vi "main_interface.vi"() -> ()   [LabVIEW 2019]
uses:
  <vilib>/Utility/miscctls.llb/LVPositionTypeDef.ctl
  <vilib>/DAQmx/read.llb/DAQmx Read (Analog 2D DBL NChan NSamp).vi
  <vilib>/DAQmx/miscellaneous.llb/DAQmx Fill In Error Info.vi
  <vilib>/Utility/file.llb/Write Delimited Spreadsheet (DBL).vi
  <vilib>/DAQmx/configure/timing.llb/DAQmx Timing (Sample Clock).vi
  <resource>/objmgr/daqmx.rc
panel:
  out "Actual Sample Rate":dbl=1000.0 format="%0.2f"
  in  "Sample Rate":dbl=3000.0
  in  "task/channels in":refnum<k21>="ADQUIRE"
  in  "PosProcessamento Button":bool
  out "Status Bar":string
  in  "Variaveis Button":bool
  in  "Home Button":bool
  in  "Calibracao Button":bool
  in  "[ESC]":bool
  in  "Tab Main":T1(tab)
  in  "Graph-PlotView-All":bool
  in  "Graph-PlotView-C":bool
  in  "Graph-PlotView-Pressoes":bool
  in  "Nome do Arquivo":string
  out "NI on?":bool
  in  "Start NI":bool
  out "aquisicao?":bool
  in  "Tempo Aquisicao":dbl
  in  "Start Aquisition":bool
  out "Dados NI [mA*10^-3]":dbl[](array[numeric])
  out "Pressoes [kPa]":dbl[](array[numeric])
  out "C Graph":dbl[][](graph)
  in  "calib_save_new":bool
  out "calib_max_atual P 11":dbl
  out "calib_min_atual P 11":dbl
  out "calib_max_atual P 10":dbl
  out "calib_min_atual P 10":dbl
  out "calib_max_atual P 9":dbl
  out "calib_min_atual P 9":dbl
  out "calib_max_atual P 8":dbl
  out "calib_min_atual P 8":dbl
  out "calib_max_atual P 7":dbl
  out "calib_min_atual P 7":dbl
  out "calib_max_atual P 6":dbl
  out "calib_min_atual P 6":dbl
  out "calib_max_atual P 5":dbl
  out "calib_min_atual P 5":dbl
  out "calib_max_atual P 4":dbl
  out "calib_min_atual P 4":dbl
  out "calib_max_atual P 3":dbl
  out "calib_min_atual P 3":dbl
  out "calib_max_atual P 2":dbl
  out "calib_min_atual P 2":dbl
  out "calib_max_atual P 1":dbl
  out "calib_min_atual P 1":dbl
  in  "calib_max_new P9":dbl
  in  "calib_min_new P9":dbl
  in  "calib_max_new P8":dbl
  in  "calib_min_new P8":dbl
  in  "calib_max_new P7":dbl
  in  "calib_min_new P7":dbl
  in  "calib_max_new P6":dbl
  in  "calib_min_new P6":dbl
  in  "calib_max_new P5":dbl
  in  "calib_min_new P5":dbl
  in  "calib_max_new P4":dbl
  in  "calib_min_new P4":dbl
  in  "calib_max_new P11":dbl
  in  "calib_min_new P11":dbl
  in  "calib_max_new P10":dbl
  in  "calib_min_new P10":dbl
  in  "calib_max_new P3":dbl
  in  "calib_min_new P3":dbl
  in  "calib_max_new P2":dbl
  in  "calib_min_new P2":dbl
  in  "calib_max_new P1":dbl
  in  "calib_min_new P1":dbl
  out "dat files":string[](array[string])
  in  "Open Folder DAT":bool
  in  "posProcessamento_button_all":bool
  in  "posProcessamento_button_indv":bool
  in  "Read TDMS file":bool
  in  "path_posProcessamento":path
  out "size dat dir":i64
  in  "Tempo aux":dbl
  out "Tempo Decorrido":dbl
  in  "Brilho do botao NI":bool
  # "Adquiri \nLazyWave"
  # "Tempo de Aquisição [s]"
  # "*Dados coletados diretamente da placa NI,\npodem estar fora de escala"
  # "Calibração atual"
  # "Nova calibração"
  # "P1"
  # "P2"
  # "P3"
  # "P4"
  # "P5"
  # "P6"
  # "P7"
  # "P8"
  # "P9"
  # "P10"
  # "P11"
  # "Arquivos processados"
  # "Processamento de um arquivo"
  # "Abrir arquivo TDMS"
  # "Abrir pasta com os arquivos .DAT"
  # "Processar todos os arquivos"
  # "Directory size"
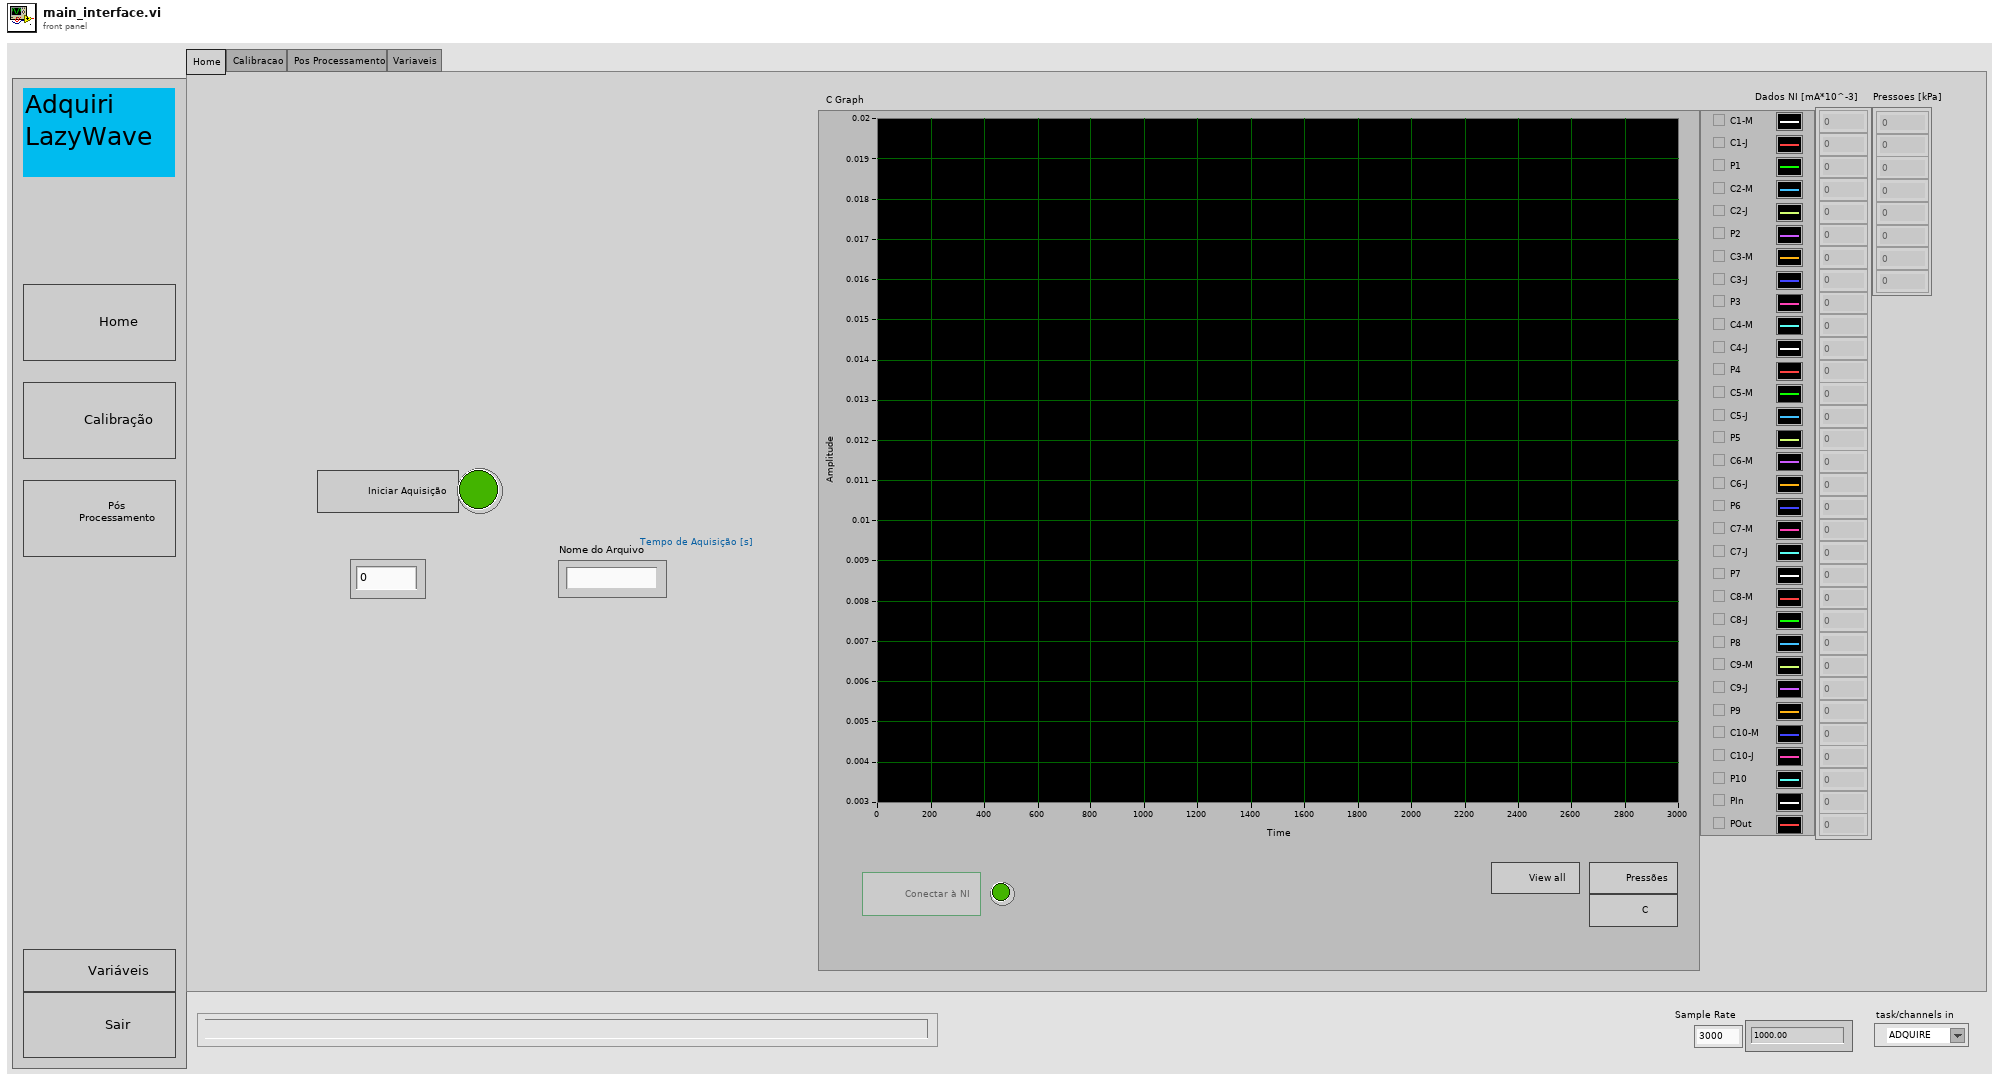
[diagram p1: front panel]
types:
  T1 = enum32{"Home", "Calibracao", "Pos Processamento", "Variaveis"}
  T2 = enum8{"Enabled", "Disabled", "Disabled and Grayed Out"}
  T3 = typedef "LVPositionTypeDef.ctl" = cluster{"Left":i32, "Top":i32}
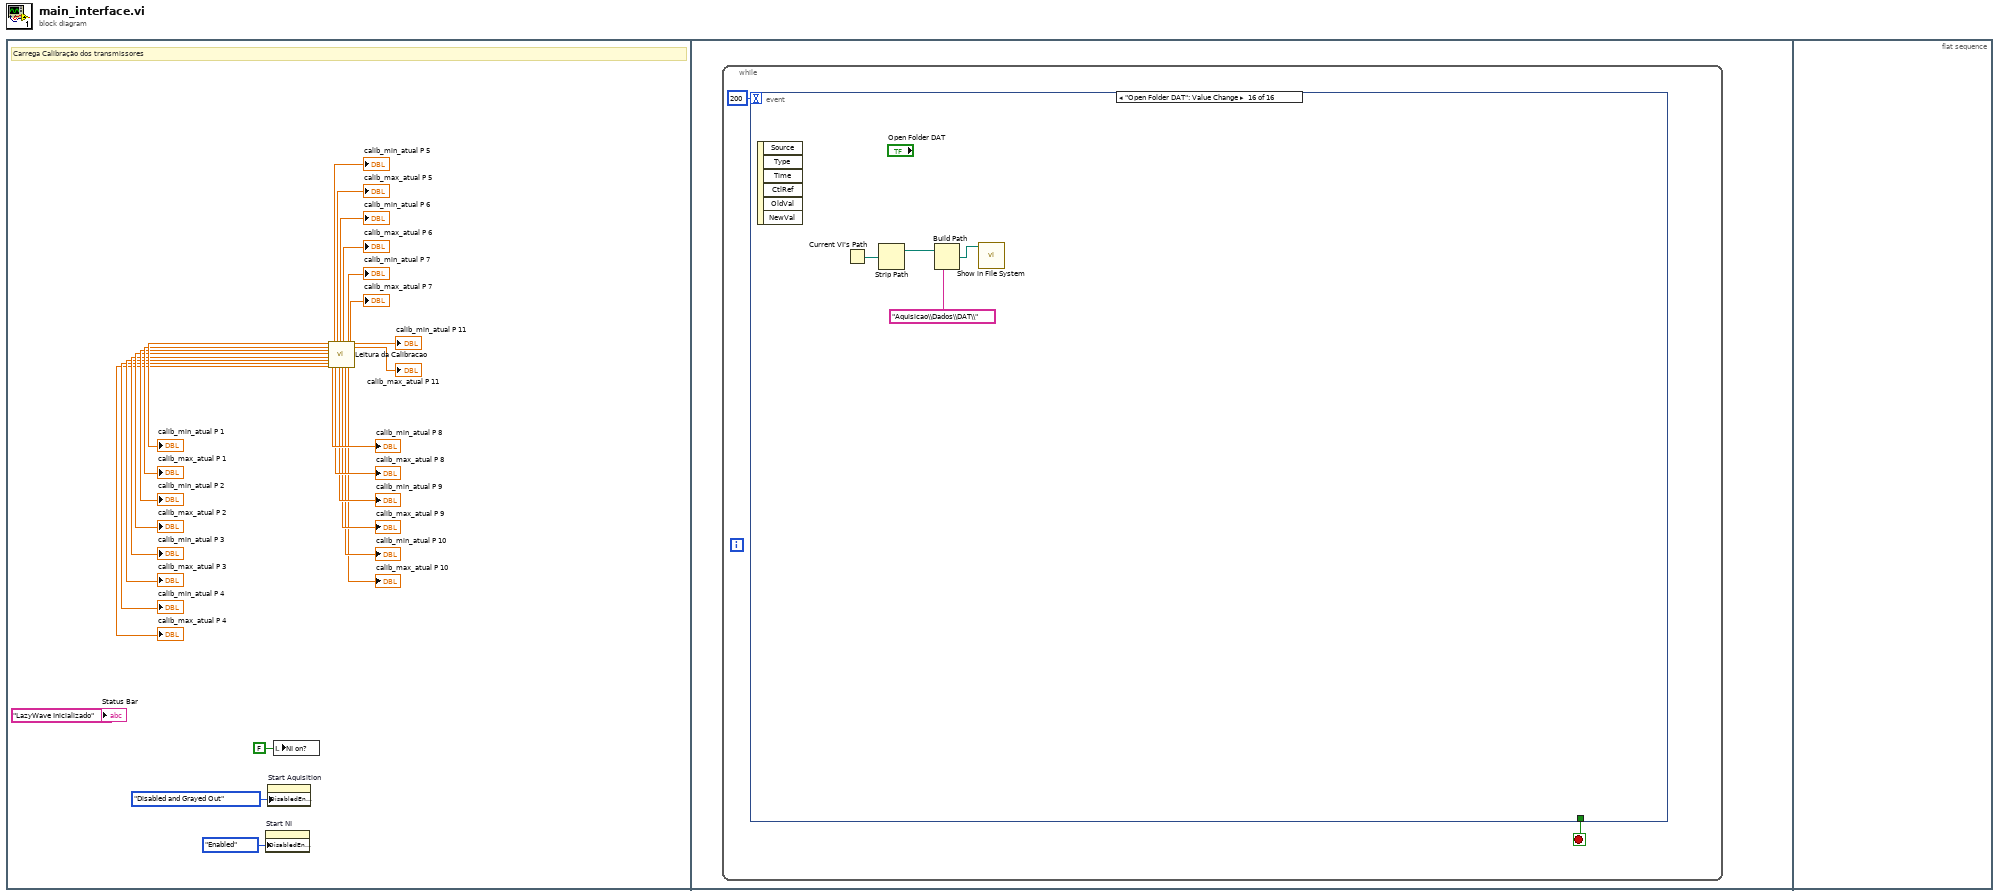
[diagram p0: block diagram]
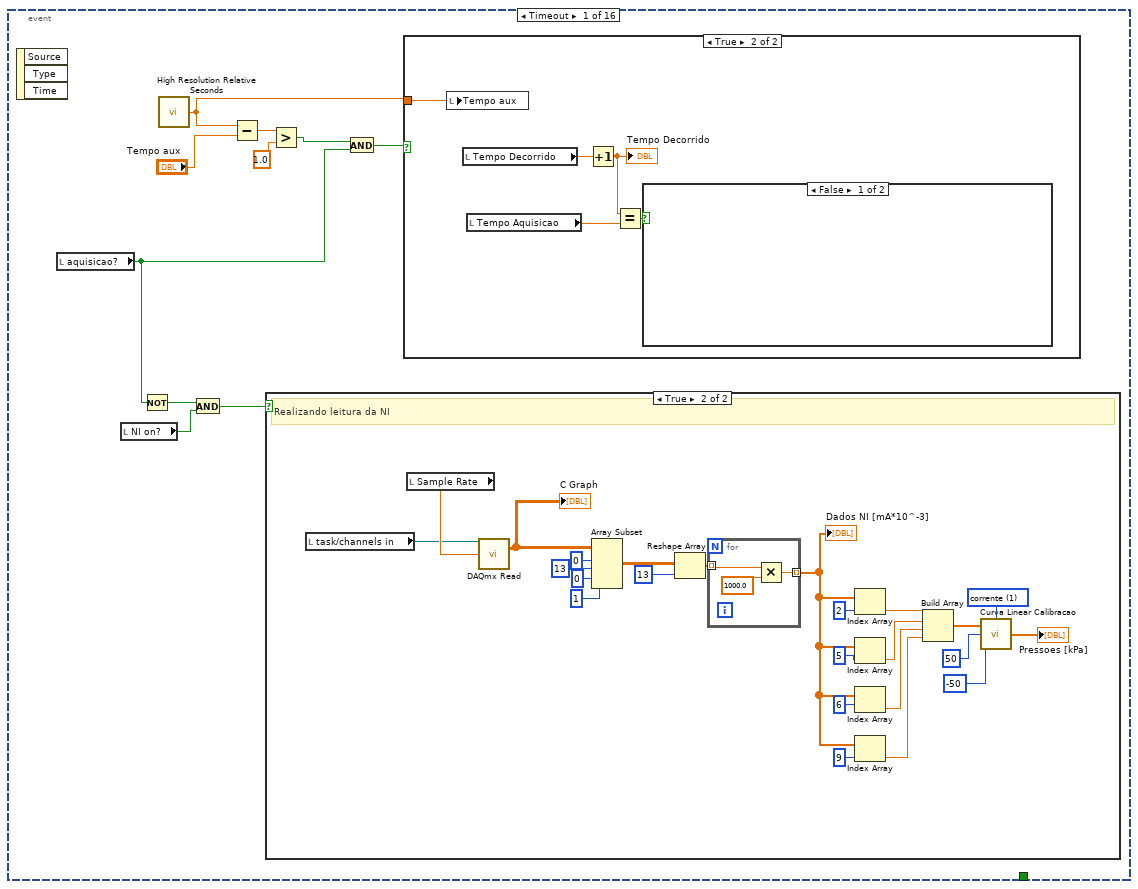
[diagram p2: hidden frame]
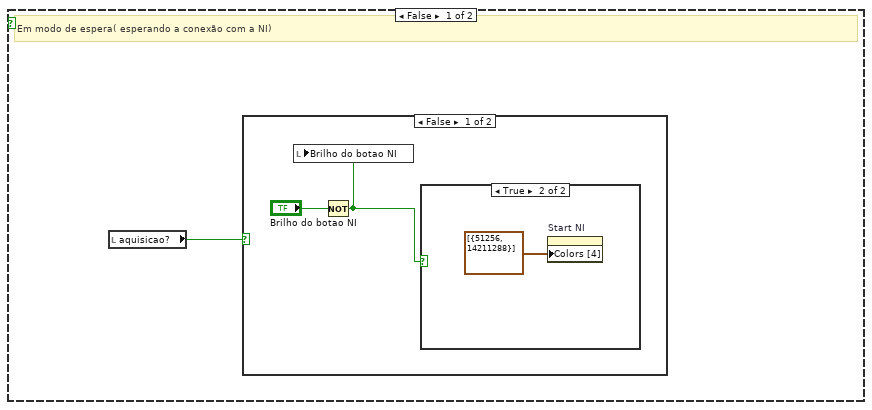
[diagram p3: hidden frame]
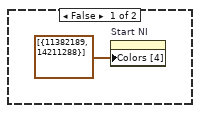
[diagram p4: hidden frame]
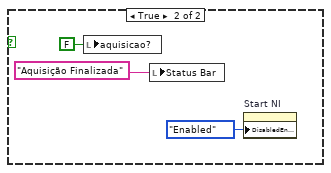
[diagram p7: hidden frame]
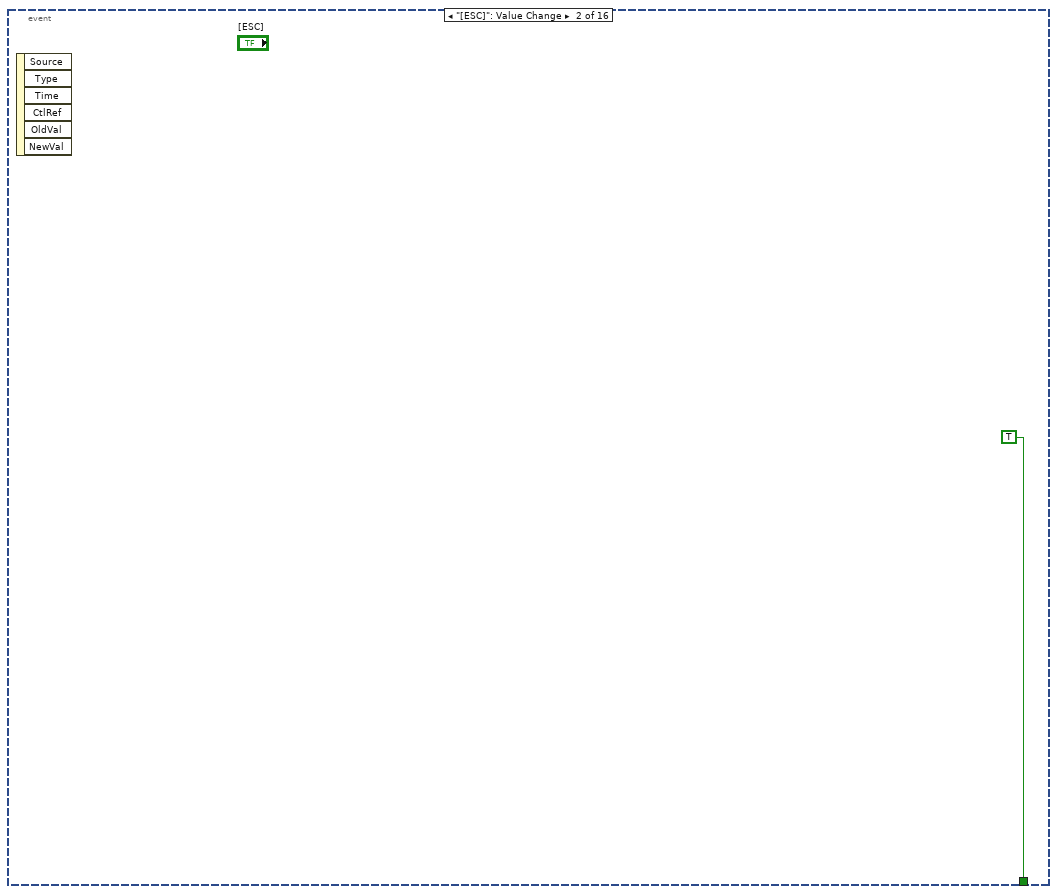
[diagram p8: hidden frame]
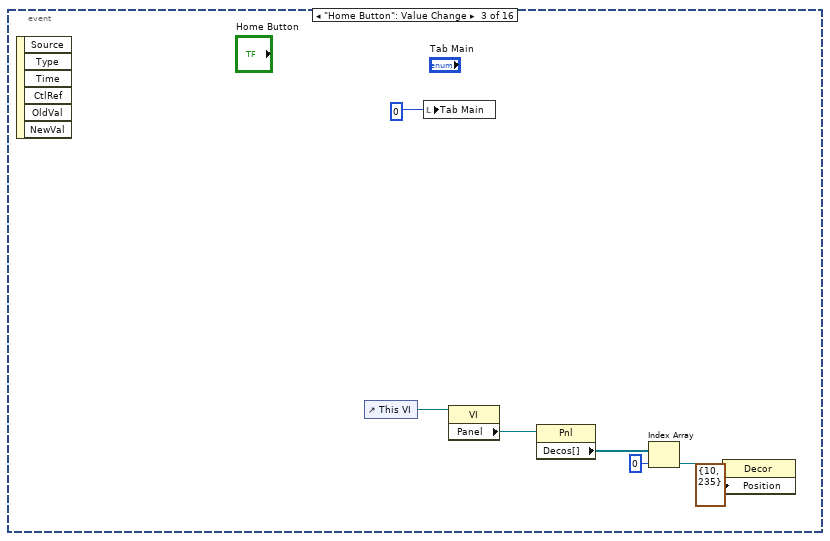
[diagram p9: hidden frame]
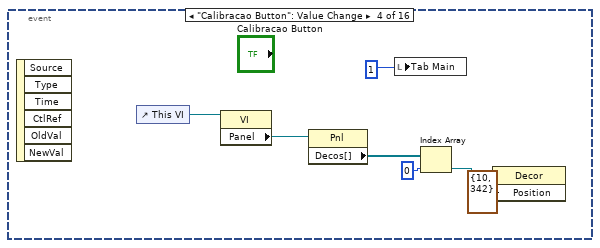
[diagram p10: hidden frame]
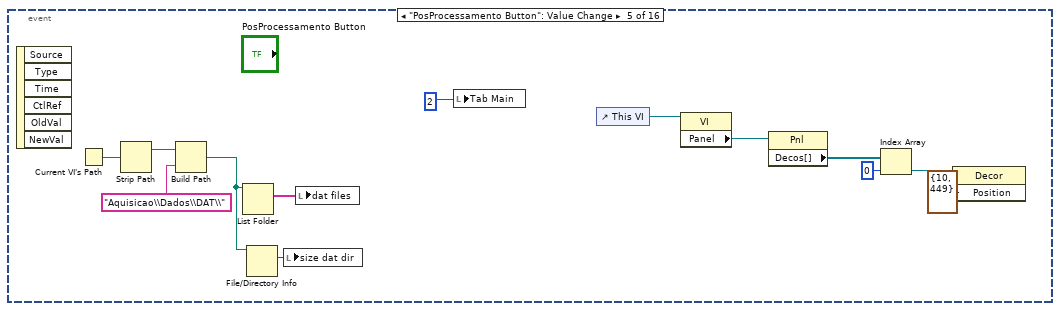
[diagram p11: hidden frame]
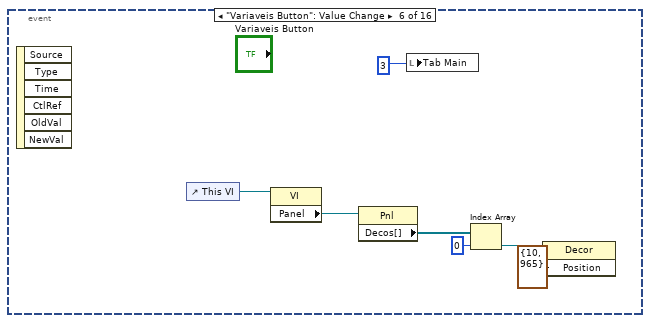
[diagram p12: hidden frame]
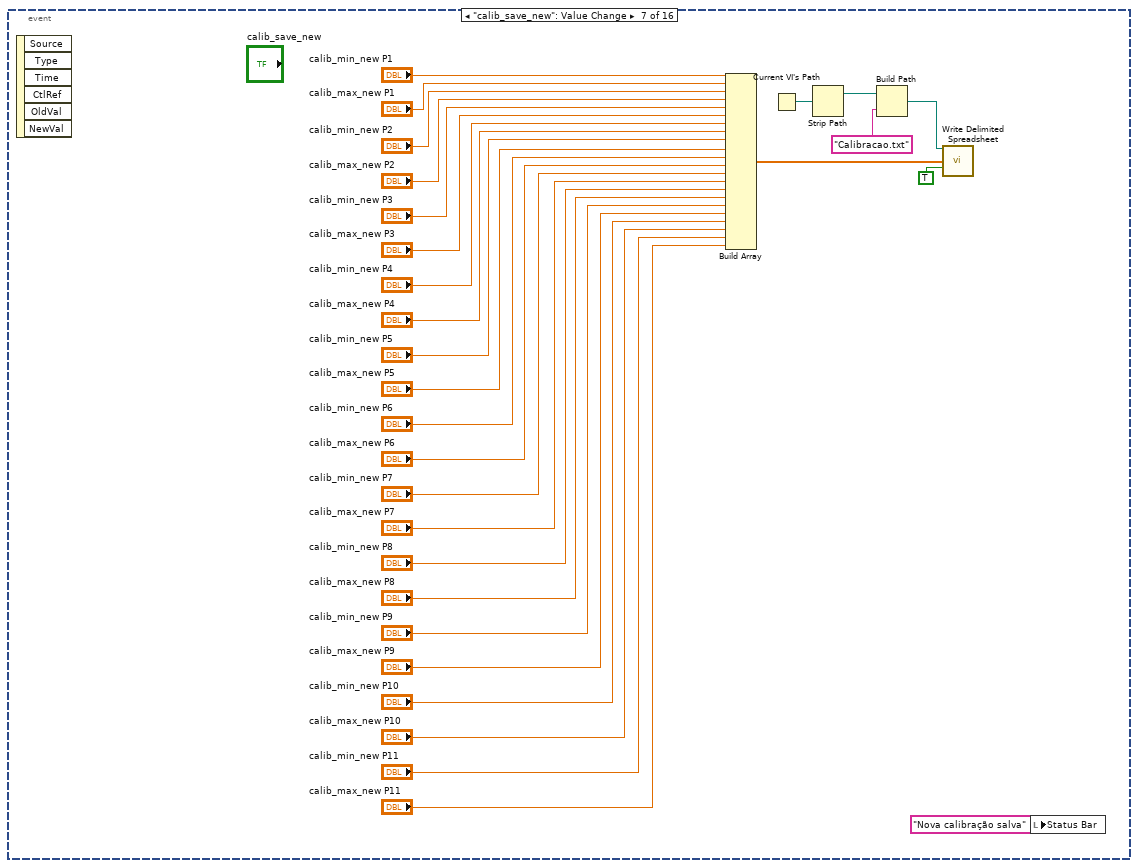
[diagram p13: hidden frame]
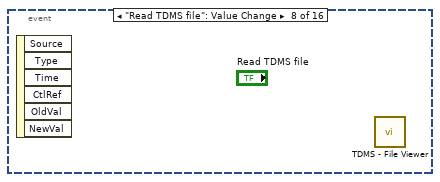
[diagram p14: hidden frame]
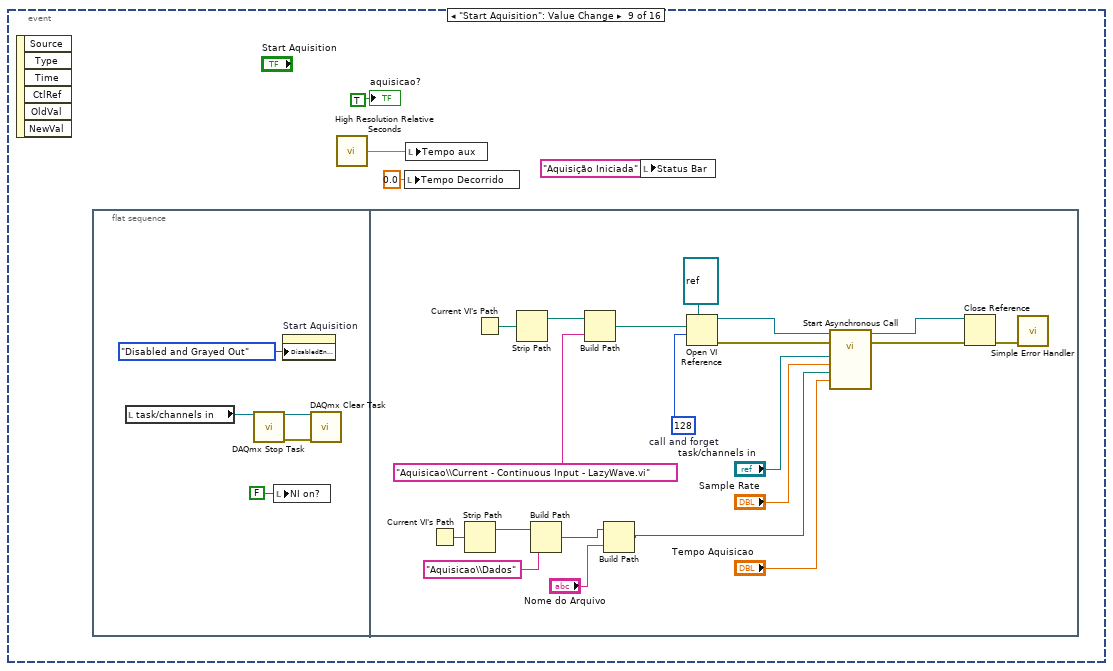
[diagram p15: hidden frame]
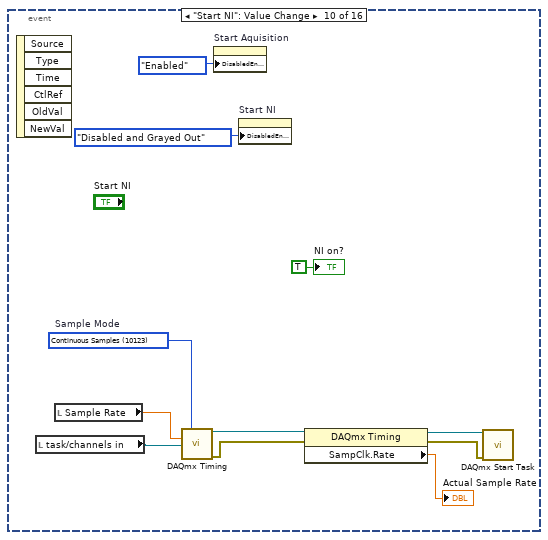
[diagram p16: hidden frame]
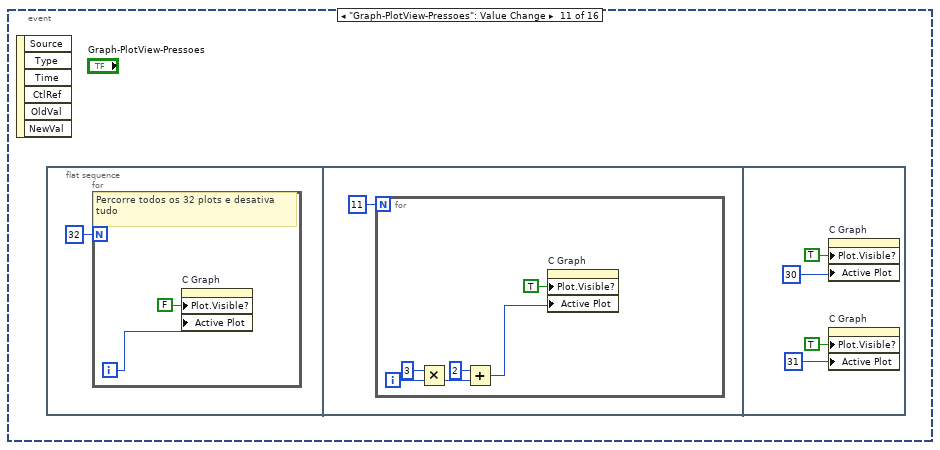
[diagram p17: hidden frame]
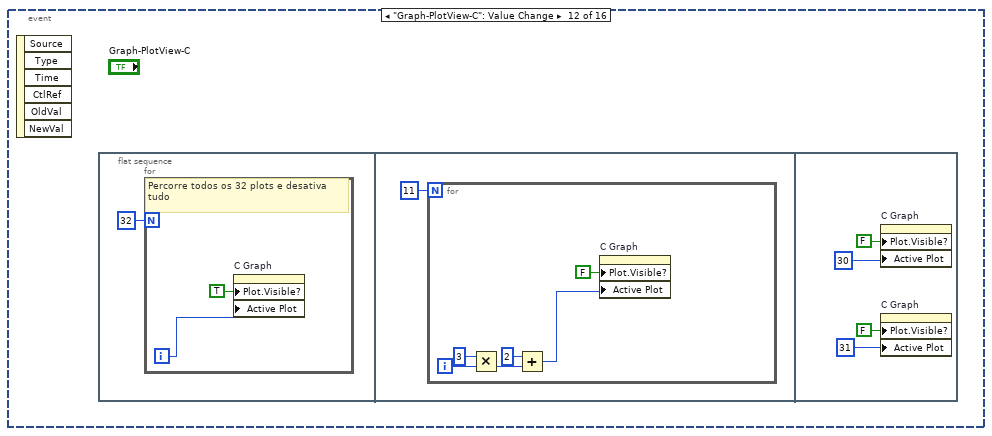
[diagram p18: hidden frame]
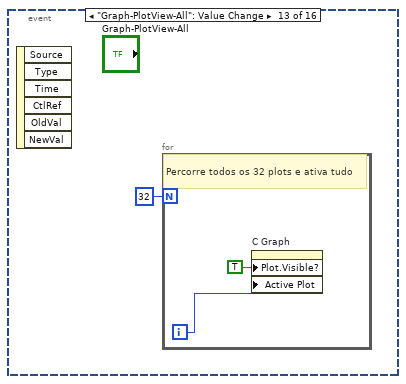
[diagram p19: hidden frame]
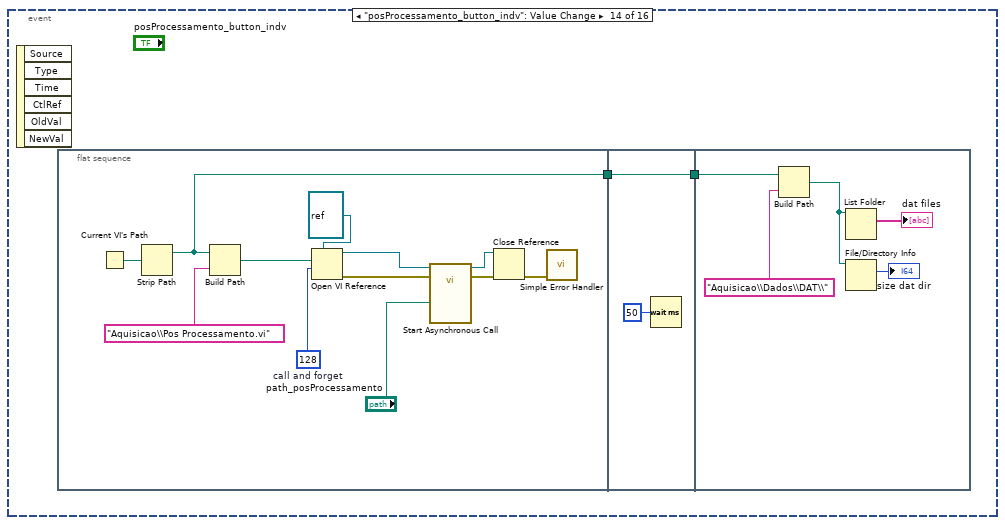
[diagram p20: hidden frame]
diagram:
  n1 = flat-sequence {
    frame #0 {
      # "Carrega Calibração dos transmissores"
      n2 = property on="Start NI" class="Bool"("DisabledEnum"=T2."Enabled" ("Disabled")) -> ()  [unwired: 2 in, 2 out]
      n3 = property on="Start Aquisition" class="Bool"("DisabledEnum"=T2."Disabled and Grayed Out" ("Disabled")) -> ()  [unwired: 2 in, 2 out]
      n4 = local write "NI on?"(FALSE ("NI on?")) -> ()
      n5 = call "Leitura da Calibracao.vi"() -> ("min P 1"=→"calib_min_atual P 1":dbl, "max P 1"=→"calib_max_atual P 1":dbl, "min P 2"=→"calib_min_atual P 2":dbl, "max P 2"=→"calib_max_atual P 2":dbl, "min P 3"=→"calib_min_atual P 3":dbl, "max P 3"=→"calib_max_atual P 3":dbl, "min P 4"=→"calib_min_atual P 4":dbl, "max P 4"=→"calib_max_atual P 4":dbl, "min P 5"=→"calib_min_atual P 5":dbl, "min P 8"=→"calib_min_atual P 8":dbl, "max P 5"=→"calib_max_atual P 5":dbl, "max P 8"=→"calib_max_atual P 8":dbl, "min P 6"=→"calib_min_atual P 6":dbl, "min P 9"=→"calib_min_atual P 9":dbl, "max P 6"=→"calib_max_atual P 6":dbl, "max P 9"=→"calib_max_atual P 9":dbl, "min P 7"=→"calib_min_atual P 7":dbl, "min P 10"=→"calib_min_atual P 10":dbl, "max P 7"=→"calib_max_atual P 7":dbl, "max P 10"=→"calib_max_atual P 10":dbl, "min P 11"=→"calib_min_atual P 11":dbl, "max P 11"=→"calib_max_atual P 11":dbl)  [unwired: 6 in]
      "Status Bar" <- "LazyWave Inicializado" ("Status Bar")
    }
    frame #1 {
      n6 = while {
        stop <- w28 stop-if-true
        n7 = event shown="[15] \"Open Folder DAT\": Value Change" {
          selector: _ -> [_ _ _ _ _ _ _ _ _ _ _ _ _ _ _ _]
          dyn-events: _ -> [_ _ _ _ _ _ _ _ _ _ _ _ _ _ _ _]
          timeout: 200 -> [_ _ _ _ _ _ _ _ _ _ _ _ _ _ _ _]
          tunnel: [_ TRUE _ _ _ _ _ _ _ _ _ _ _ _ _ _] -> w28
          event Timeout {
            n8 = event-data() -> ()  [unwired: 1 in, 3 out]
            n9 = local read "aquisicao?"() -> (w32:bool)
            n10 = local read "NI on?"() -> (w31:bool)
            n11 = Not(x=w32) -> (.not. x?=w30:bool)
            n12 = call <vilib>:"High Resolution Relative Seconds.vi"() -> ("relative seconds"=w35:dbl)
            n13 = And(x=w30, y=w31) -> (x .and. y?=w29:bool)
            n14 = Subtract(x=w35, y="Tempo aux") -> (x-y=w37:dbl)
            n15 = case shown="True" w29 {
              frame False {
                # "Em modo de espera( esperando a conexão com a NI)"
                n16 = local read "aquisicao?"() -> (w39:bool)
                n17 = case shown="False" w39 {
                  frame False {
                    n18 = Not(x="Brilho do botao NI") -> (.not. x?=w40:bool)
                    n19 = local write "Brilho do botao NI"(w40) -> ()
                    n20 = case shown="True" w40 {
                      frame False {
                        n21 = property on="Start NI" class="Bool"("Colors [4]"=cluster{u32, u32}[] [{11382189, 14211288}]) -> ()  [unwired: 2 in, 2 out]
                      }
                      frame True {
                        n22 = property on="Start NI" class="Bool"("Colors [4]"=cluster{u32, u32}[] [{51256, 14211288}]) -> ()  [unwired: 2 in, 2 out]
                      }
                    }
                  }
                  frame True {
                  }
                }
              }
              frame True {
                w47 = u16 1 items=["tensao", "corrente"] ("input type")
                # "Realizando leitura da NI"
                n23 = local read "task/channels in"() -> (w66:refnum<k21>)
                n24 = local read "Sample Rate"() -> (w67:dbl)
                n25 = call-poly <vilib>:"DAQmx Read.vi"("task/channels in"=w66, "number of samples per channel"=w67) -> ("data"=w65:dbl[][])  [unwired: 11 in, 2 out]
                "C Graph" <- w65
                n26 = Array Subset(array=w65, index (row)=0 ("index"), length (row)=13 ("length"), index (col)=0 ("index"), length (col)=1 ("length")) -> (w60:dbl[][])
                n27 = Reshape Array(w60, 13 ("dimension size")) -> (w58:dbl[])
                n28 = for {
                  tunnel: w58 -> [w70] mode=indexing
                  tunnel: [w68] -> w53 mode=indexing
                  n29 = Multiply(x=w70, y=1000.0) -> (x*y=w68:dbl)
                }
                "Dados NI [mA*10^-3]" <- w53
                n30 = Index Array(array=w53, index=2) -> (element=w52:dbl)
                n31 = Index Array(array=w53, index=5) -> (element=w51:dbl)
                n32 = Index Array(array=w53, index=6) -> (element=w50:dbl)
                n33 = Index Array(array=w53, index=9) -> (element=w49:dbl)
                n34 = Build Array(w52, w51, w50, w49) -> (w48:dbl[])
                n35 = call "Curva Linear Calibracao.vi"("input type"=w47, "MIN"=-50, "MAX"=50, "input"=w48) -> ("output"=→"Pressoes [kPa]":dbl[])
              }
            }
            n36 = Greater?(x=w37, y=1.0) -> (0:w33:bool)
            n37 = And(x=w33, y=w32) -> (x .and. y?=w34:bool)
            n38 = case shown="True" w34 {
              tunnel: w35 -> [_ w74]
              frame False {
              }
              frame True {
                n39 = local write "Tempo aux"(w74) -> ()
                n40 = local read "Tempo Decorrido"() -> (w75:dbl)
                n41 = local read "Tempo Aquisicao"() -> (w71:dbl)
                n42 = Increment(x=w75) -> (x+1=w72:dbl)
                "Tempo Decorrido" <- w72
                n43 = Equal?(x=w72, y=w71) -> (x = y?=w73:bool)
                n44 = case shown="False" w73 {
                  frame False {
                  }
                  frame True {
                    n45 = local write "aquisicao?"(FALSE ("aquisicao?")) -> ()
                    n46 = local write "Status Bar"("Aquisição Finalizada" ("String")) -> ()
                    n47 = property on="Start NI" class="Bool"("DisabledEnum"=T2."Enabled" ("Disabled")) -> ()  [unwired: 2 in, 2 out]
                  }
                }
              }
            }
          }
          event "[ESC]": Value Change {
            n48 = event-data() -> ()  [unwired: 1 in, 6 out]
          }
          event "Home Button": Value Change {
            n49 = event-data() -> ()  [unwired: 1 in, 6 out]
            n50 = control-ref of="This VI"() -> (w85:refnum<vi>)
            n51 = local write "Tab Main"(0) -> ()
            n52 = property class="VI"(reference=w85) -> ("Panel"=w84:refnum<vi>)  [unwired: 1 in, 2 out]
            n53 = property class="Pnl"(reference=w84) -> ("Decos[]"=w83:refnum<vi>[])  [unwired: 1 in, 2 out]
            n54 = Index Array(array=w83, index=0) -> (element=w81:refnum<vi>)
            n55 = property class="Decor"(reference=w81, "Position"=T3 {"Left"=10, "Top"=235}) -> ()  [unwired: 1 in, 2 out]
          }
          event "Calibracao Button": Value Change {
            n56 = event-data() -> ()  [unwired: 1 in, 6 out]
            n57 = control-ref of="This VI"() -> (w92:refnum<vi>)
            n58 = property class="VI"(reference=w92) -> ("Panel"=w91:refnum<vi>)  [unwired: 1 in, 2 out]
            n59 = property class="Pnl"(reference=w91) -> ("Decos[]"=w90:refnum<vi>[])  [unwired: 1 in, 2 out]
            n60 = local write "Tab Main"(1) -> ()
            n61 = Index Array(array=w90, index=0) -> (element=w89:refnum<vi>)
            n62 = property class="Decor"(reference=w89, "Position"=T3 {"Left"=10, "Top"=342}) -> ()  [unwired: 1 in, 2 out]
          }
          event "PosProcessamento Button": Value Change {
            n63 = event-data() -> ()  [unwired: 1 in, 6 out]
            n64 = Current VI's Path() -> (path=w98:path)
            n65 = Strip Path(path=w98) -> (stripped path=w99:path)  [unwired: 1 out]
            n66 = Build Path(base path=w99, name or relative path="Aquisicao\\Dados\\DAT\\") -> (appended path=w94:path)
            n67 = List Folder(path=w94) -> (filenames=w96:string[])  [unwired: 3 in, 3 out]
            n68 = File/Directory Info(path=w94) -> (size=w95:i64)  [unwired: 1 in, 6 out]
            n69 = local write "size dat dir"(w95) -> ()
            n70 = local write "dat files"(w96) -> ()
            n71 = local write "Tab Main"(2) -> ()
            n72 = control-ref of="This VI"() -> (w105:refnum<vi>)
            n73 = property class="VI"(reference=w105) -> ("Panel"=w104:refnum<vi>)  [unwired: 1 in, 2 out]
            n74 = property class="Pnl"(reference=w104) -> ("Decos[]"=w103:refnum<vi>[])  [unwired: 1 in, 2 out]
            n75 = Index Array(array=w103, index=0) -> (element=w102:refnum<vi>)
            n76 = property class="Decor"(reference=w102, "Position"=T3 {"Left"=10, "Top"=449}) -> ()  [unwired: 1 in, 2 out]
          }
          event "Variaveis Button": Value Change {
            n77 = event-data() -> ()  [unwired: 1 in, 6 out]
            n78 = control-ref of="This VI"() -> (w112:refnum<vi>)
            n79 = property class="VI"(reference=w112) -> ("Panel"=w111:refnum<vi>)  [unwired: 1 in, 2 out]
            n80 = property class="Pnl"(reference=w111) -> ("Decos[]"=w110:refnum<vi>[])  [unwired: 1 in, 2 out]
            n81 = local write "Tab Main"(3) -> ()
            n82 = Index Array(array=w110, index=0) -> (element=w109:refnum<vi>)
            n83 = property class="Decor"(reference=w109, "Position"=T3 {"Left"=10, "Top"=965}) -> ()  [unwired: 1 in, 2 out]
          }
          event "calib_save_new": Value Change {
            n84 = event-data() -> ()  [unwired: 1 in, 6 out]
            n85 = Build Array("calib_min_new P1", "calib_max_new P1", "calib_min_new P2", "calib_max_new P2", "calib_min_new P3", "calib_max_new P3", "calib_min_new P4", "calib_max_new P4", "calib_min_new P5", "calib_max_new P5", "calib_min_new P6", "calib_max_new P6", "calib_min_new P7", "calib_max_new P7", "calib_min_new P8", "calib_max_new P8", "calib_min_new P9", "calib_max_new P9", "calib_min_new P10", "calib_max_new P10", "calib_min_new P11", "calib_max_new P11") -> (w139:dbl[])
            n86 = Current VI's Path() -> (path=w140:path)
            n87 = Strip Path(path=w140) -> (stripped path=w141:path)  [unwired: 1 out]
            n88 = Build Path(base path=w141, name or relative path="Calibracao.txt") -> (appended path=w142:path)
            n89 = call-poly <vilib>:"Write Delimited Spreadsheet.vi"("file path (dialog if empty)"=w142, "1D data"=w139, "append to file? (new file:F)"=TRUE) -> ()  [unwired: 11 in, 2 out]
            n90 = local write "Status Bar"("Nova calibração salva" ("String")) -> ()
          }
          event "Read TDMS file": Value Change {
            n91 = event-data() -> ()  [unwired: 1 in, 6 out]
            n92 = call <vilib>:"TDMS - File Viewer.vi"() -> ()  [unwired: 6 in, 2 out]
          }
          event "Start Aquisition": Value Change {
            n93 = event-data() -> ()  [unwired: 1 in, 6 out]
            n94 = flat-sequence {
              frame #0 {
                n95 = local read "task/channels in"() -> (w151:refnum<k21>)
                n96 = call <vilib>:"DAQmx Stop Task.vi"("task/channels in"=w151) -> ("task out"=w149:refnum<k21>, "error out"=w150:errorcluster)  [unwired: 13 in]
                n97 = local write "NI on?"(FALSE ("NI on?")) -> ()
                n98 = property on="Start Aquisition" class="Bool"("DisabledEnum"=T2."Disabled and Grayed Out" ("Disabled")) -> ()  [unwired: 2 in, 2 out]
                n99 = call <vilib>:"DAQmx Clear Task.vi"("task in"=w149, "error in"=w150) -> ()  [unwired: 13 in, 1 out]
              }
              frame #1 {
                w171 = 128  # call and forget
                n100 = Current VI's Path() -> (path=w156:path)
                n101 = Strip Path(path=w156) -> (stripped path=w155:path)  [unwired: 1 out]
                n102 = Current VI's Path() -> (path=w164:path)
                n103 = Strip Path(path=w164) -> (stripped path=w163:path)  [unwired: 1 out]
                n104 = Build Path(base path=w155, name or relative path="Aquisicao\\Dados") -> (appended path=w154:path)
                n105 = Build Path(base path=w163, name or relative path="Aquisicao\\Current - Continuous Input - LazyWave.vi") -> (appended path=w161:path)
                n106 = Build Path(base path=w154, name or relative path="Nome do Arquivo") -> (appended path=w152:path)
                n107 = Open VI Reference(type specifier VI Refnum (for type only)=refnum<vi> refnum, vi path=w161, options=w171) -> (vi reference=w169:refnum<vi>, error out=w168:errorcluster)  [unwired: 3 in]
                n108 = call-by-ref "Start Asynchronous Call"(reference=w169, error in=w168, "Tempo Aquisicao"="Tempo Aquisicao", "TDMS File Path"=w152, "Sample Rate"="Sample Rate", "task/channels in"="task/channels in") -> (reference out=w166:refnum<vi>, error out=w167:errorcluster)  [unwired: 8 in]
                n109 = Close Reference(reference=w166, error in (no error)=w167) -> (error out=w165:errorcluster)
                n110 = call <vilib>:"Simple Error Handler.vi"("error in (no error)"=w165) -> ()  [unwired: 4 in, 5 out]
              }
            }
            n111 = call <vilib>:"High Resolution Relative Seconds.vi"() -> ("relative seconds"=w145:dbl)
            n112 = local write "Tempo Decorrido"(0.0 ("Tempo Decorrido")) -> ()
            n113 = local write "Tempo aux"(w145) -> ()
            n114 = local write "Status Bar"("Aquisição Iniciada" ("String")) -> ()
            "aquisicao?" <- TRUE ("aquisicao?")
          }
          event "Start NI": Value Change {
            w176 = 10123 items=["Finite Samples"=10178, "Continuous Samples"=10123, "Hardware Timed Single Point"=12522]  # Sample Mode
            n115 = event-data() -> ()  [unwired: 1 in, 6 out]
            n116 = local read "task/channels in"() -> (w179:refnum<k21>)
            n117 = local read "Sample Rate"() -> (w180:dbl)
            n118 = call-poly <vilib>:"DAQmx Timing.vi"("task/channels in"=w179, "sample mode"=w176, "rate"=w180) -> ("task out"=w178:refnum<k21>, "error out"=w177:errorcluster)  [unwired: 11 in]
            n119 = property on="Start Aquisition" class="Bool"("DisabledEnum"=T2."Enabled" ("Disabled")) -> ()  [unwired: 2 in, 2 out]
            n120 = property on="Start NI" class="Bool"("DisabledEnum"=T2."Disabled and Grayed Out" ("Disabled")) -> ()  [unwired: 2 in, 2 out]
            n121 = property class="DAQmx Timing"(reference=w178, error in=w177) -> (reference out=w181:refnum<k21>, error out=w182:errorcluster, "SampClk.Rate"=→"Actual Sample Rate":dbl)
            n122 = call <vilib>:"DAQmx Start Task.vi"("task/channels in"=w181, "error in"=w182) -> ()  [unwired: 12 in, 2 out]
            "NI on?" <- TRUE ("NI on?")
          }
          event "Graph-PlotView-Pressoes": Value Change {
            n123 = event-data() -> ()  [unwired: 1 in, 6 out]
            n124 = flat-sequence {
              frame #0 {
                n125 = for {
                  N: 32 -> [_]
                  i -> [w184]
                  # "Percorre todos os 32 plots e desativa tudo"
                  n126 = property on="C Graph" class="WFGraph (strict)"("Plot.Visible?"=FALSE ("Plot.Visible"), "Active Plot"=w184) -> ()  [unwired: 2 in, 2 out]
                }
              }
              frame #1 {
                n127 = for {
                  N: 11 -> [_]
                  i -> [w192]
                  n128 = Multiply(x=3, y=w192) -> (x*y=w190:i32)
                  n129 = Add(x=2, y=w190) -> (x+y=w187:i32)
                  n130 = property on="C Graph" class="WFGraph (strict)"("Plot.Visible?"=TRUE ("Plot.Visible"), "Active Plot"=w187) -> ()  [unwired: 2 in, 2 out]
                }
              }
              frame #2 {
                n131 = property on="C Graph" class="WFGraph (strict)"("Plot.Visible?"=TRUE ("Plot.Visible"), "Active Plot"=u32 30) -> ()  [unwired: 2 in, 2 out]
                n132 = property on="C Graph" class="WFGraph (strict)"("Plot.Visible?"=TRUE ("Plot.Visible"), "Active Plot"=u32 31) -> ()  [unwired: 2 in, 2 out]
              }
            }
          }
          event "Graph-PlotView-C": Value Change {
            n133 = event-data() -> ()  [unwired: 1 in, 6 out]
            n134 = flat-sequence {
              frame #0 {
                n135 = for {
                  N: 32 -> [_]
                  i -> [w198]
                  # "Percorre todos os 32 plots e desativa tudo"
                  n136 = property on="C Graph" class="WFGraph (strict)"("Plot.Visible?"=TRUE ("Plot.Visible"), "Active Plot"=w198) -> ()  [unwired: 2 in, 2 out]
                }
              }
              frame #1 {
                n137 = for {
                  N: 11 -> [_]
                  i -> [w206]
                  n138 = Multiply(x=3, y=w206) -> (x*y=w204:i32)
                  n139 = Add(x=2, y=w204) -> (x+y=w201:i32)
                  n140 = property on="C Graph" class="WFGraph (strict)"("Plot.Visible?"=FALSE ("Plot.Visible"), "Active Plot"=w201) -> ()  [unwired: 2 in, 2 out]
                }
              }
              frame #2 {
                n141 = property on="C Graph" class="WFGraph (strict)"("Plot.Visible?"=FALSE ("Plot.Visible"), "Active Plot"=u32 30) -> ()  [unwired: 2 in, 2 out]
                n142 = property on="C Graph" class="WFGraph (strict)"("Plot.Visible?"=FALSE ("Plot.Visible"), "Active Plot"=u32 31) -> ()  [unwired: 2 in, 2 out]
              }
            }
          }
          event "Graph-PlotView-All": Value Change {
            n143 = event-data() -> ()  [unwired: 1 in, 6 out]
            n144 = for {
              N: 32 -> [_]
              i -> [w212]
              # "Percorre todos os 32 plots e ativa tudo"
              n145 = property on="C Graph" class="WFGraph (strict)"("Plot.Visible?"=TRUE ("Plot.Visible"), "Active Plot"=w212) -> ()  [unwired: 2 in, 2 out]
            }
          }
          event "posProcessamento_button_indv": Value Change {
            n146 = event-data() -> ()  [unwired: 1 in, 6 out]
            n147 = flat-sequence {
              tunnel: [w216] -> w215
              tunnel: w215 -> [w229]
              tunnel: [w229] -> w214
              tunnel: w214 -> [w233]
              frame #0 {
                w218 = 128  # call and forget
                n148 = Current VI's Path() -> (path=w222:path)
                n149 = Strip Path(path=w222) -> (stripped path=w216:path)  [unwired: 1 out]
                n150 = Build Path(base path=w216, name or relative path="Aquisicao\\Pos Processamento.vi") -> (appended path=w221:path)
                n151 = Open VI Reference(type specifier VI Refnum (for type only)=refnum<vi> refnum, vi path=w221, options=w218) -> (vi reference=w227:refnum<vi>, error out=w226:errorcluster)  [unwired: 3 in]
                n152 = call-by-ref "Start Asynchronous Call"(reference=w227, error in=w226, "file path"="path_posProcessamento") -> (reference out=w224:refnum<vi>, error out=w225:errorcluster)  [unwired: 1 in]
                n153 = Close Reference(reference=w224, error in (no error)=w225) -> (error out=w223:errorcluster)
                n154 = call <vilib>:"Simple Error Handler.vi"("error in (no error)"=w223) -> ()  [unwired: 4 in, 5 out]
              }
              frame #1 {
                n155 = Wait (ms)(milliseconds to wait=u32 50) -> ()  [unwired: 1 out]
              }
              frame #2 {
                n156 = Build Path(base path=w233, name or relative path="Aquisicao\\Dados\\DAT\\") -> (appended path=w231:path)
                n157 = List Folder(path=w231) -> (filenames=→"dat files":string[])  [unwired: 3 in, 3 out]
                n158 = File/Directory Info(path=w231) -> (size=→"size dat dir":i64)  [unwired: 1 in, 6 out]
              }
            }
          }
          event "posProcessamento_button_all": Value Change {
            n159 = event-data() -> ()  [unwired: 1 in, 6 out]
            n160 = flat-sequence {
              tunnel: [w239] -> w236
              tunnel: w236 -> [w251]
              tunnel: [w251] -> w235
              tunnel: w235 -> [w252]
              frame #0 {
                w240 = 128  # call and forget
                n161 = Current VI's Path() -> (path=w244:path)
                n162 = Strip Path(path=w244) -> (stripped path=w239:path)  [unwired: 1 out]
                n163 = Build Path(base path=w239, name or relative path="Aquisicao\\main Pos Processamento.vi") -> (appended path=w243:path)
                n164 = Build Path(base path=w239, name or relative path="Aquisicao\\Dados") -> (appended path=w237:path)
                n165 = Open VI Reference(type specifier VI Refnum (for type only)=refnum<vi> refnum, vi path=w243, options=w240) -> (vi reference=w249:refnum<vi>, error out=w248:errorcluster)  [unwired: 3 in]
                n166 = call-by-ref "Start Asynchronous Call"(reference=w249, error in=w248, "path"=w237) -> (reference out=w246:refnum<vi>, error out=w247:errorcluster)  [unwired: 1 in]
                n167 = Close Reference(reference=w246, error in (no error)=w247) -> (error out=w245:errorcluster)
                n168 = call <vilib>:"Simple Error Handler.vi"("error in (no error)"=w245) -> ()  [unwired: 4 in, 5 out]
              }
              frame #1 {
                n169 = Wait (ms)(milliseconds to wait=u32 50) -> ()  [unwired: 1 out]
              }
              frame #2 {
                n170 = Build Path(base path=w252, name or relative path="Aquisicao\\Dados\\DAT\\") -> (appended path=w254:path)
                n171 = call <vilib>:"Show in File System.vi"("file or directory path"=w254) -> ()  [unwired: 10 in, 1 out]
              }
            }
          }
          event "Open Folder DAT": Value Change {
            n172 = event-data() -> ()  [unwired: 1 in, 6 out]
            n173 = Current VI's Path() -> (path=w258:path)
            n174 = Strip Path(path=w258) -> (stripped path=w257:path)  [unwired: 1 out]
            n175 = Build Path(base path=w257, name or relative path="Aquisicao\\Dados\\DAT\\") -> (appended path=w255:path)
            n176 = call <vilib>:"Show in File System.vi"("file or directory path"=w255) -> ()  [unwired: 10 in, 1 out]
          }
        }
      }
    }
    frame #2 {
    }
  }
